vi "ErrorHandler.vi"(8 "error in (no error)":errorcluster, 11 "MessageQueue":refnum<queue>) -> (0 "error out":errorcluster, 3 "MessageQueue":refnum<queue>)   [LabVIEW 2017, in "FlagImpairModule.lvlib"]
uses:
  FlagImpairModule.lvlib
  PublicAPI/Arguments/Messages/clMessage.ctl
panel:
  in  "Message (Error)":string="Error"
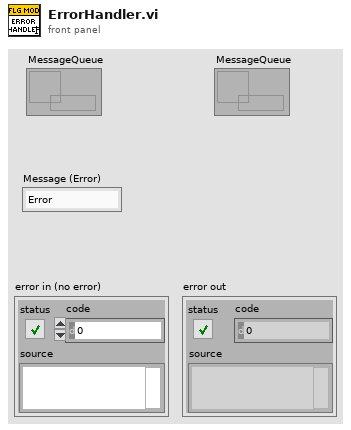
[diagram p1: front panel]
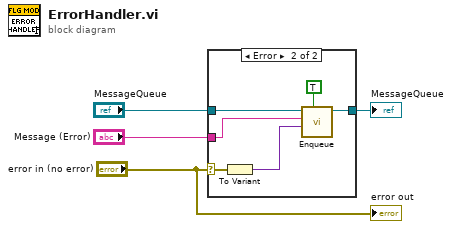
[diagram p0: block diagram]
diagram:
  n1 = case shown="Error" "error in (no error)" {
    selector: "error in (no error)" -> [_ w10]
    tunnel: [w5 w7] -> w2
    tunnel: "MessageQueue" -> [w5 w11]
    tunnel: "Message (Error)" -> [_ w8]
    frame No Error {
    }
    frame Error {
      n2 = To Variant(anything=w10) -> (Variant=w9:variant)
      n3 = call "Enqueue.vi"("Priority (F)"=TRUE, "Message Data"=w9, "Message"=w8, "MessageQueue"=w11) -> ("MessageQueue"=w7:refnum<queue>)  [unwired: 6 in, 1 out]
    }
  }
  "MessageQueue" <- w2
  "error out" <- "error in (no error)"
